vi "TestLIDAR.vi"() -> ()   [LabVIEW 2009]
panel:
  out "Dot Prod":dbl
  out "Points of Intersection":cluster{dbl, dbl}[](array[cluster])
  in  "Obstacle":cluster{"x":dbl, "y":dbl}={"x"=2.0, "y"=0.0}
  in  "Vector Bearing":dbl=0.1
  in  "Obstacle Radius":dbl=0.1
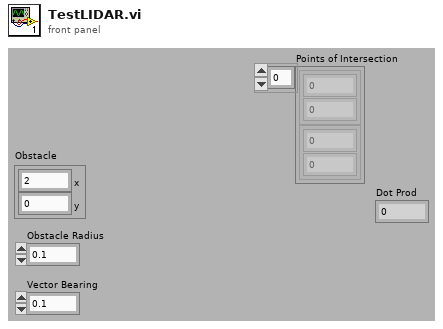
[diagram p1: front panel]
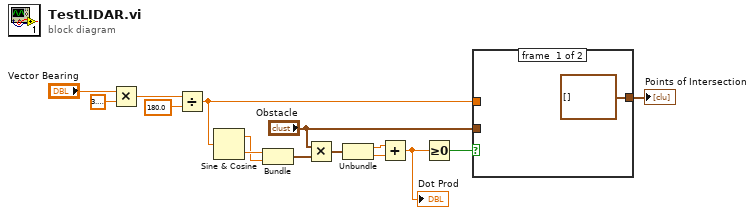
[diagram p0: block diagram]
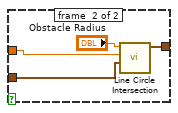
[diagram p2: hidden frame]
diagram:
  n1 = Multiply(x="Vector Bearing", y=3.141592653589793) -> (x*y=w13:dbl)
  n2 = Divide(x=w13, y=180.0) -> (x/y=w10:dbl)
  n3 = Sine & Cosine(0:w10) -> (1:w8:dbl, 2:w9:dbl)
  n4 = Bundle(w9, w8) -> (w7:cluster{dbl, dbl})  [unwired: 1 in]
  n5 = Multiply(x="Obstacle", y=w7) -> (x*y=w5:cluster{dbl, dbl})
  n6 = Unbundle(w5) -> (w4:dbl, w3:dbl)
  n7 = Add(x=w4, y=w3) -> (x+y=w2:dbl)
  "Dot Prod" <- w2
  n8 = Greater Or Equal To 0?(x=w2) -> (x >= 0?=w1:bool)
  n9 = case shown="False" w1 {
    tunnel: [cluster{dbl, dbl}[] [] ("Points of Intersection") w19] -> w11
    tunnel: w10 -> [_ w18]
    tunnel: "Obstacle" -> [_ w17]
    frame #0 {
    }
    frame #1 {
      n10 = call "Line Circle Intersection.vi"("Circle Center"=w17, "Line's Angle (rads)"=w18, "Circle Radius"="Obstacle Radius") -> ("Points of Intersection"=w19:cluster{dbl, dbl}[])  [unwired: 6 in, 2 out]
    }
  }
  "Points of Intersection" <- w11
